vi "SaveML.vi"(6 "error in":errorcluster, 7 "Nom de la sequence":string, 8 "line":string, 9 "color win":u32(colorbox), 10 "color loose":u32(colorbox), 11 "Pos":cluster{string[], string[]}[](array[cluster])) -> (0 "error out":errorcluster, 2 "script ML":string)   [LabVIEW 2021]
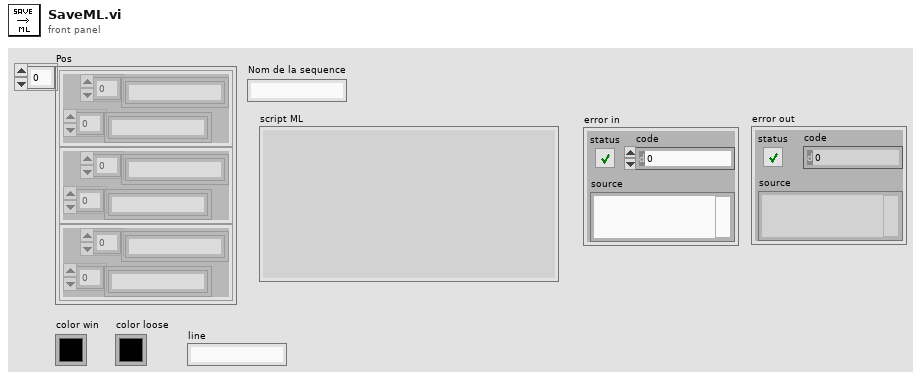
[diagram p1: front panel]
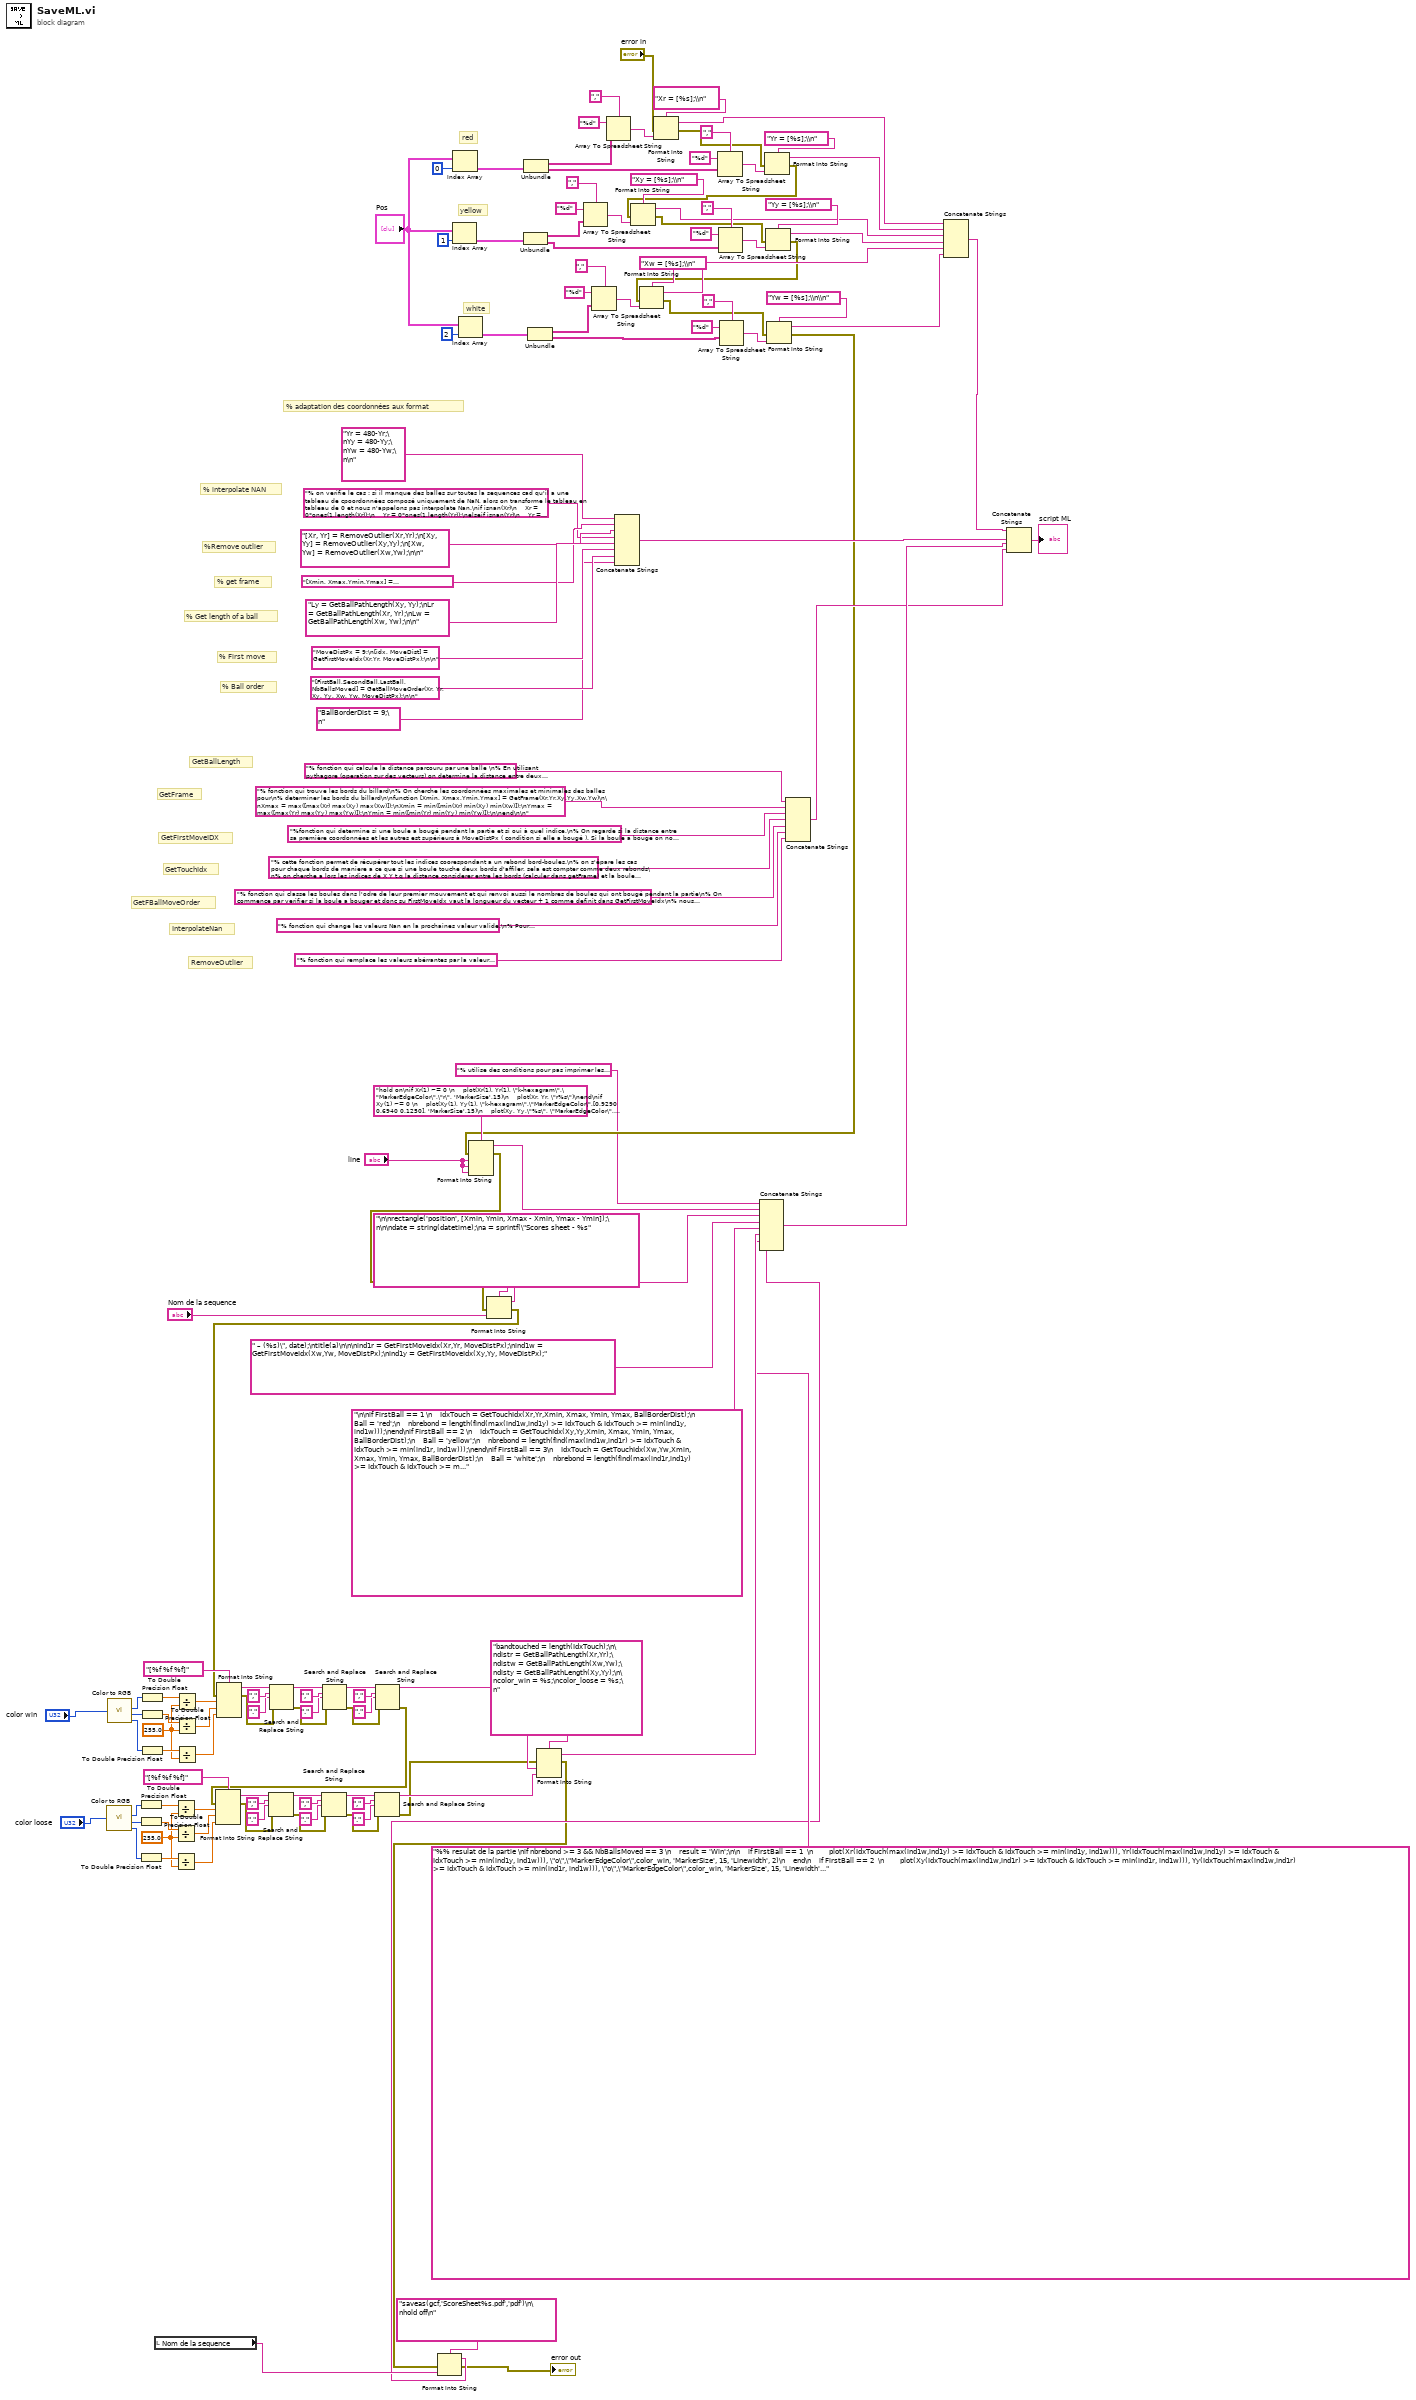
[diagram p0: block diagram]
diagram:
  w44 = 255.0
  w67 = 255.0
  # "RemoveOutlier"
  # "InterpolateNan"
  # "GetFBallMoveOrder"
  # "GetTouchIdx"
  # "GetFirstMoveIDX"
  # "GetFrame"
  # "GetBallLength"
  # "white"
  # "yellow"
  # "red"
  # "% Ball order"
  # "% First move"
  # "% Get length of a ball"
  # "% get frame"
  # "%Remove outlier"
  # "% interpolate NAN"
  # "% adaptation des coordonnées aux format"
  n1 = call <vilib>:"Color to RGB.vi"("Color"="color loose") -> ("R"=w50:u8, "G"=w49:u8, "B"=w48:u8)  [unwired: 1 out]
  n2 = call <vilib>:"Color to RGB.vi"("Color"="color win") -> ("R"=w73:u8, "G"=w72:u8, "B"=w71:u8)  [unwired: 1 out]
  n3 = To Double Precision Float(number=w50) -> (double precision float=w47:dbl)
  n4 = To Double Precision Float(number=w49) -> (double precision float=w46:dbl)
  n5 = To Double Precision Float(number=w48) -> (double precision float=w45:dbl)
  n6 = To Double Precision Float(number=w73) -> (double precision float=w70:dbl)
  n7 = To Double Precision Float(number=w72) -> (double precision float=w69:dbl)
  n8 = To Double Precision Float(number=w71) -> (double precision float=w68:dbl)
  n9 = local read "Nom de la sequence"() -> (w9:string)
  n10 = Divide(x=w47, y=w44) -> (x/y=w43:dbl)
  n11 = Divide(x=w46, y=w44) -> (x/y=w42:dbl)
  n12 = Divide(x=w45, y=w44) -> (x/y=w41:dbl)
  n13 = Divide(x=w70, y=w67) -> (x/y=w66:dbl)
  n14 = Divide(x=w69, y=w67) -> (x/y=w65:dbl)
  n15 = Divide(x=w68, y=w67) -> (x/y=w64:dbl)
  n16 = Index Array(array="Pos", index=1) -> (element=w136:cluster{string[], string[]})
  n17 = Index Array(array="Pos", index=0) -> (element=w137:cluster{string[], string[]})
  n18 = Index Array(array="Pos", index=2) -> (element=w135:cluster{string[], string[]})
  n19 = Unbundle(w136) -> (w120:string[], w106:string[])
  n20 = Unbundle(w137) -> (w134:string[], w126:string[])
  n21 = Unbundle(w135) -> (w107:string[], w105:string[])
  n22 = Array To Spreadsheet String(delimiter (Tab)=",", array=w120, 3:"%d" ("format string")) -> (spreadsheet string=w122:string)
  n23 = Array To Spreadsheet String(delimiter (Tab)=",", array=w107, 3:"%d" ("format string")) -> (spreadsheet string=w113:string)
  n24 = Array To Spreadsheet String(delimiter (Tab)=",", array=w134, 3:"%d" ("format string")) -> (spreadsheet string=w131:string)
  n25 = Concatenate Strings("Yr = 480-Yr;\nYy = 480-Yy;\nYw = 480-Yw;\n\n", "[Xmin, Xmax,Ymin,Ymax] = GetFrame(Xr,Yr,Xy,Yy,Xw,Yw);\n\n", "[Xr, Yr] = RemoveOutlier(Xr,Yr);\n[Xy, Yy] = RemoveOutlier(Xy,Yy);\n[Xw, Yw] = RemoveOutlier(Xw,Yw);\n\n", "% on verifie le cas : si il manque des balles sur toutes la sequences cad qu'il a une tableau de cpoordonnées composé uniquement de NaN, alors on transforme le tableau en tableau de 0 et nous n'appelons pas interpolate Nan.\nif isnan(Xr)\n    Xr = 0*ones(1,length(Xr));\n    Yr = 0*ones(1,length(Yr));\nelseif isnan(Yr)\n    Yr = 0*ones(1,length(Yr));\n    Xr = 0*ones(1,length(Xr));\nelse\n    [Xr, Yr] = InterpolateNan(Xr,Yr);\nend\n\nif isnan(Xy)\n    Xy = 0*ones(1,length(Xy));\n    Yy = 0*ones(1,length(Yy));\nelseif isnan(Yy)\n    Yy = 0*ones(1,length(Yy));\n    Xy = 0*ones(1,length(Xy));\nelse\n    [Xy, Yy] = InterpolateNan(Xy,Yy);\nend\n\nif isnan(Xw)\n    Xw = 0*ones(1,length(Xw));\n    Yw = 0*ones(1,length(Yw));\nelseif isnan(Yw)\n    Yw = 0*ones(1,length(Yw));\n    Xw = 0*ones(1,length(Xw));\nelse\n    [Xw, Yw] = InterpolateNan(Xw,Yw);\nend\n\n", "Ly = GetBallPathLength(Xy, Yy);\nLr = GetBallPathLength(Xr, Yr);\nLw = GetBallPathLength(Xw, Yw);\n\n", "MoveDistPx = 9;\n[idx, MoveDist] = GetFirstMoveIdx(Xr,Yr, MoveDistPx);\n\n", "[FirstBall,SecondBall,LastBall, NbBallsMoved] = GetBallMoveOrder(Xr, Yr, Xy, Yy, Xw, Yw, MoveDistPx);\n\n", "BallBorderDist = 9;\n") -> (w77:string)
  n26 = Format Into String(format string="Xr = [%s];\\n", error in="error in", w131) -> (resulting string=w87:string, error out=w25:errorcluster)  [unwired: 1 in]
  n27 = Array To Spreadsheet String(delimiter (Tab)=",", array=w126, 3:"%d" ("format string")) -> (spreadsheet string=w127:string)
  n28 = Array To Spreadsheet String(delimiter (Tab)=",", array=w106, 3:"%d" ("format string")) -> (spreadsheet string=w117:string)
  n29 = Array To Spreadsheet String(delimiter (Tab)=",", array=w105, 3:"%d" ("format string")) -> (spreadsheet string=w109:string)
  n30 = Format Into String(format string="Yr = [%s];\\n", error in=w25, w127) -> (resulting string=w104:string, error out=w24:errorcluster)  [unwired: 1 in]
  n31 = Format Into String(format string="Xy = [%s];\\n", error in=w24, w122) -> (resulting string=w103:string, error out=w23:errorcluster)  [unwired: 1 in]
  n32 = Format Into String(format string="Yy = [%s];\\n", error in=w23, w117) -> (resulting string=w102:string, error out=w22:errorcluster)  [unwired: 1 in]
  n33 = Format Into String(format string="Xw = [%s];\\n", error in=w22, w113) -> (resulting string=w101:string, error out=w21:errorcluster)  [unwired: 1 in]
  n34 = Format Into String(format string="Yw = [%s];\\n\\n", error in=w21, w109) -> (resulting string=w100:string, error out=w20:errorcluster)  [unwired: 1 in]
  n35 = Format Into String(format string="hold on\nif Xr(1) ~= 0 \n    plot(Xr(1), Yr(1), \"k-hexagram\",\"MarkerEdgeColor\",\"r\", 'MarkerSize',15)\n    plot(Xr, Yr, \"r%s\")\nend\nif Xy(1) ~= 0 \n    plot(Xy(1), Yy(1), \"k-hexagram\",\"MarkerEdgeColor\",[0.9290 0.6940 0.1250], 'MarkerSize',15)\n    plot(Xy, Yy,\"%s\", \"MarkerEdgeColor\", [0.9290 0.6940 0.1250])\nend\nif Xw(1) ~= 0 \n    plot(Xw(1), Yw(1), \"k-hexagram\",\"MarkerEdgeColor\",\"b\", 'MarkerSize',15)\n    plot(Xw, Yw, \"b%s\")\nend\n", error in=w20, "line", "line", "line") -> (resulting string=w81:string, error out=w19:errorcluster)  [unwired: 1 in]
  n36 = Format Into String(format string="\n\nrectangle('position', [Xmin, Ymin, Xmax - Xmin, Ymax - Ymin]);\n\n\ndate = string(datetime);\na = sprintf(\"Scores sheet - %s", error in=w19, "Nom de la sequence") -> (resulting string=w80:string, error out=w18:errorcluster)  [unwired: 1 in]
  n37 = Format Into String(format string="[%f %f %f]", error in=w18, w66, w65, w64) -> (resulting string=w63:string, error out=w17:errorcluster)  [unwired: 1 in]
  n38 = Search and Replace String(input string=w63, search string=",", replace string="." ("replace string (\"\")"), error in=w17) -> (result string=w56:string, error out=w16:errorcluster)  [unwired: 4 in, 2 out]
  n39 = Search and Replace String(input string=w56, search string=",", replace string="." ("replace string (\"\")"), error in=w16) -> (result string=w55:string, error out=w15:errorcluster)  [unwired: 4 in, 2 out]
  n40 = Search and Replace String(input string=w55, search string=",", replace string="." ("replace string (\"\")"), error in=w15) -> (result string=w54:string, error out=w14:errorcluster)  [unwired: 4 in, 2 out]
  n41 = Format Into String(format string="[%f %f %f]", error in=w14, w43, w42, w41) -> (resulting string=w40:string, error out=w13:errorcluster)  [unwired: 1 in]
  n42 = Search and Replace String(input string=w40, search string=",", replace string="." ("replace string (\"\")"), error in=w13) -> (result string=w33:string, error out=w12:errorcluster)  [unwired: 4 in, 2 out]
  n43 = Search and Replace String(input string=w33, search string=",", replace string="." ("replace string (\"\")"), error in=w12) -> (result string=w32:string, error out=w11:errorcluster)  [unwired: 4 in, 2 out]
  n44 = Search and Replace String(input string=w32, search string=",", replace string="." ("replace string (\"\")"), error in=w11) -> (result string=w31:string, error out=w10:errorcluster)  [unwired: 4 in, 2 out]
  n45 = Format Into String(format string="bandtouched = length(IdxTouch);\n\ndistr = GetBallPathLength(Xr,Yr);\ndistw = GetBallPathLength(Xw,Yw);\ndisty = GetBallPathLength(Xy,Yy);\n\ncolor_win = %s;\ncolor_loose = %s;\n", error in=w10, w54, w31) -> (resulting string=w30:string, error out=w6:errorcluster)  [unwired: 1 in]
  n46 = Format Into String(format string="saveas(gcf,'ScoreSheet%s.pdf','pdf')\n\nhold off\n", error in=w6, w9) -> (resulting string=w7:string, error out=→"error out":errorcluster)  [unwired: 1 in]
  n47 = Concatenate Strings("% utilise des conditions pour pas imprimer les coordonnées si la boule n'est pas la donc que sa coordonnées en X soit egale a 0\n", w81, w80, " – (%s)\", date);\ntitle(a)\n\n\nind1r = GetFirstMoveIdx(Xr,Yr, MoveDistPx);\nind1w = GetFirstMoveIdx(Xw,Yw, MoveDistPx);\nind1y = GetFirstMoveIdx(Xy,Yy, MoveDistPx);", "\n\nif FirstBall == 1 \n    IdxTouch = GetTouchIdx(Xr,Yr,Xmin, Xmax, Ymin, Ymax, BallBorderDist);\n    Ball = 'red';\n    nbrebond = length(find(max(ind1w,ind1y) >= IdxTouch & IdxTouch >= min(ind1y, ind1w)));\nend\nif FirstBall == 2 \n    IdxTouch = GetTouchIdx(Xy,Yy,Xmin, Xmax, Ymin, Ymax, BallBorderDist);\n    Ball = 'yellow';\n    nbrebond = length(find(max(ind1w,ind1r) >= IdxTouch & IdxTouch >= min(ind1r, ind1w)));\nend\nif FirstBall == 3\n    IdxTouch = GetTouchIdx(Xw,Yw,Xmin, Xmax, Ymin, Ymax, BallBorderDist);\n    Ball = 'white';\n    nbrebond = length(find(max(ind1r,ind1y) >= IdxTouch & IdxTouch >= min(ind1y, ind1r)));\nend\n", w30, "%% resulat de la partie \nif nbrebond >= 3 && NbBallsMoved == 3 \n    result = 'Win';\n\n    if FirstBall == 1  \n        plot(Xr(IdxTouch(max(ind1w,ind1y) >= IdxTouch & IdxTouch >= min(ind1y, ind1w))), Yr(IdxTouch(max(ind1w,ind1y) >= IdxTouch & IdxTouch >= min(ind1y, ind1w))), \"o\",\"MarkerEdgeColor\",color_win, 'MarkerSize', 15, 'Linewidth', 2)\n    end\n    if FirstBall == 2  \n        plot(Xy(IdxTouch(max(ind1w,ind1r) >= IdxTouch & IdxTouch >= min(ind1r, ind1w))), Yy(IdxTouch(max(ind1w,ind1r) >= IdxTouch & IdxTouch >= min(ind1r, ind1w))), \"o\",\"MarkerEdgeColor\",color_win, 'MarkerSize', 15, 'Linewidth', 2)\n    end\n    if FirstBall == 3\n        plot(Xw(IdxTouch(max(ind1r,ind1y) >= IdxTouch & IdxTouch >= min(ind1y, ind1r))), Yw(IdxTouch(max(ind1r,ind1y) >= IdxTouch & IdxTouch >= min(ind1y, ind1r))), \"o\",\"MarkerEdgeColor\",color_win, 'MarkerSize', 15, 'Linewidth', 2)\n    end\n\nelse \n    result = 'Loose';\n\n    if FirstBall == 1  \n        plot(Xr(IdxTouch), Yr(IdxTouch), \"o\",\"MarkerEdgeColor\",color_loose, 'MarkerSize', 15,  'Linewidth', 2)\n    end\n    if FirstBall == 2  \n        plot(Xy(IdxTouch), Yy(IdxTouch), \"o\",\"MarkerEdgeColor\",color_loose, 'MarkerSize', 15,  'Linewidth', 2)\n    end\n    if FirstBall == 3\n        plot(Xw(IdxTouch), Yw(IdxTouch), \"o\",\"MarkerEdgeColor\",color_loose, 'MarkerSize', 15,  'Linewidth', 2)\n    end\nend\n\n%legende \n% legend('hahahahha', 'location' , 'southeastoutside')\ntext(Xmin+20 , Ymin-10, sprintf('Score sheet for \"%s\"', Ball))\ntext(Xmin+20 , Ymin-20, sprintf('---\"%s\"---', result))\ntext(Xmin+420 , Ymin-20, sprintf('%d band(s) touched', bandtouched))\ntext(Xmin+420 , Ymin-10, sprintf('%d ball(s) moved', NbBallsMoved))\ntext(Xmin+20 , Ymin-30, sprintf('red : %.0fpx', round(distr)))\ntext(Xmin+220 , Ymin-30, sprintf('yellow : %.0f px', round(disty)))\ntext(Xmin+420 , Ymin-30, sprintf('white : %.0f px', round(distw)))\n\n \naxis off\n\n", w7) -> (w76:string)
  n48 = Concatenate Strings("% fonction qui calcule la distance parcouru par une balle \n% En utilisant pythagore (operation sur des vecteurs) on determine la distance entre deux coordonnées à l'aide de la fonction diff(X)  succésive puis on additionne ces longueurs grasse a la fct sum.\n \nfunction PathLength = GetBallPathLength(X,Y)\n\nlength_vector = sqrt(diff(X).^2 + diff(Y).^2);\nPathLength = sum(length_vector);\n\nend\n\n", "% fonction qui trouve les bords du billard\n% On cherche les coordonnées maximales et minimales des balles pour\n% determiner les bords du billard\n\nfunction [Xmin, Xmax,Ymin,Ymax] = GetFrame(Xr,Yr,Xy,Yy,Xw,Yw)\n\nXmax = max([max(Xr) max(Xy) max(Xw)]);\nXmin = min([min(Xr) min(Xy) min(Xw)]);\nYmax = max([max(Yr) max(Yy) max(Yw)]);\nYmin = min([min(Yr) min(Yy) min(Yw)]);\n\nend\n\n", "%fonction qui determine si une boule a bougé pendant la partie et si oui à quel indice.\n% On regarde si la distance entre sa première coordonnées et les autres est supérieurs à MoveDistPx ( condition si elle a bougé ). Si la boule a bougé on note l'indice de son premier mouvement dans FirstMoveIdx et la distance dans MoveDist.\n% En revanche si elle n'a pas bougé on met FirstMoveIdx au dernier indice + 1. de maniere a ce que cet indice corresponde a un indice impossible. MoveDist sera alors definit a 0.\n% De plus nous avons etudiez le cas a savoir si il manque une boule et donc que les opérations sur les vecteurs ne sont pas possibles.\nfunction [FirstMoveIdx, MoveDist] = GetFirstMoveIdx(X,Y, MoveDistPx)\nX1 = X(1);\nY1 = Y(1);\nX = X - X1;\nY = Y - Y1;\n\nif X1 == 0 && Y1 == 0\n    d = 0;\nelse\n    d = sqrt( X.^2 + Y.^2 );\nend\nif d <= MoveDistPx \n    FirstMoveIdx = length(X)+1;\n    MoveDist = 0;\nelse\n    FirstMoveIdx = find(d>MoveDistPx, 1);\n    MoveDist = sqrt(X(FirstMoveIdx).^2 + Y(FirstMoveIdx).^2);\nend\n\nend\n\n", "% cette fonction permet de récupérer tout les indices coorespondant a un rebond bord-boules.\n% on s'épare les cas pour chaque bords de maniere a ce que si une boule touche deux bords d'affiler, sela est compter comme deux rebonds\n% on cherche a lors les indices de X Y t.q la distance considerer entre les bords (calculer dans getFrame) et la boule soit inferieur ou egale a BallBorderDist.\n\nfunction [IdxTouch]=GetTouchIdx(X,Y,Xmin, Xmax, Ymin, Ymax, BallBorderDist)\n\nIdxTouch_Xmax = find( (X+BallBorderDist) >= Xmax);\nb = [0, diff(IdxTouch_Xmax)];\nIdxTouch_Xmax = IdxTouch_Xmax((b ~= 1).*IdxTouch_Xmax > 1);\n\nIdxTouch_Xmin = find( (X-BallBorderDist) <= Xmin);\nb = [0, diff(IdxTouch_Xmin)];\nIdxTouch_Xmin = IdxTouch_Xmin((b ~= 1).*IdxTouch_Xmin > 1);\n\nIdxTouch_Ymax = find( (Y+BallBorderDist) >= Ymax);\nb = [0, diff(IdxTouch_Ymax)];\nIdxTouch_Ymax = IdxTouch_Ymax((b ~= 1).*IdxTouch_Ymax > 1);\n\nIdxTouch_Ymin = find( (Y-BallBorderDist) <= Ymin);\nb = [0, diff(IdxTouch_Ymin)];\nIdxTouch_Ymin = IdxTouch_Ymin((b ~= 1).*IdxTouch_Ymin > 1);\n\nIdxTouch = sort([IdxTouch_Xmax, IdxTouch_Xmin, IdxTouch_Ymax, IdxTouch_Ymin]);\n\nend\n\n", "% fonction qui classe les boules dans l'odre de leur premier mouvement et qui renvoi aussi le nombres de boules qui ont bougé pendant la partie\n% On commence par verifier si la boule a bouger et donc su FirstMoveIdx vaut la longueur du vecteur + 1 comme definit dans GetFirstMoveIdx\n% nous cherchons donc ensuite a evaluer tout les cas possibles en commencant par chercher la plus petite de FirstMoveIdx et donc de l'appeler Firstball \n% Nous analysons ensuite la longueur de ce vecteur pour que si elle vaut 2 ou trois on comare les MoveDistPx et donc de savoir laquelle est la vrai premiere. \n% une fois que la firstball est definit, on fait de meme mais avec la plus grande Valeur de FirstMoveIdx pour definir la troisieme boules et on prossede a la meme methode que pour firstball. \n% enfin lorsque nous avons first et lastball, la deuxieme est celle qui manque et que l'on peut trouver avec la fct setdiff qui compore [lastball first ball] avec [1 2 3]\n\nfunction [FirstBall,SecondBall,LastBall, NbBallsMoved] = GetBallMoveOrder(Xr, Yr, Xy, Yy, Xw, Yw, MoveDistPx) \n\na = 3;\n\n[FirstMoveIdxr, MoveDistr] = GetFirstMoveIdx(Xr,Yr, MoveDistPx);\nif FirstMoveIdxr == length(Xr)+1\n    a = a-1;\nend\n[FirstMoveIdxy, MoveDisty] = GetFirstMoveIdx(Xy,Yy, MoveDistPx);\nif FirstMoveIdxy == length(Xy)+1\n    a = a-1;\nend\n[FirstMoveIdxw, MoveDistw] = GetFirstMoveIdx(Xw,Yw, MoveDistPx);\nif FirstMoveIdxw == length(Xw)+1\n    a = a-1;\nend\n\nNbBallsMoved = a;\n\nFirstMoveIdx = [FirstMoveIdxr, FirstMoveIdxy, FirstMoveIdxw];\nMoveDist = [MoveDistr, MoveDisty, MoveDistw];\n\nFirstBall = find(FirstMoveIdx == min(FirstMoveIdx));\n\nif length(FirstBall) == 1\n    LastBall = find(FirstMoveIdx == max(FirstMoveIdx));\n    if length(LastBall) == 2\n        LastBall = find(MoveDist == min(MoveDist(LastBall(1)), MoveDist(LastBall(2))));\n    end \nend \n\nif length(FirstBall) == 2\n    FirstBall = find(MoveDist == max(MoveDist(FirstBall(1)), MoveDist(FirstBall(2))));\n    LastBall = find(FirstMoveIdx == max(FirstMoveIdx));\nend\n\nif length(FirstBall) == 3\n    FirstBall = find(MoveDist == max(MoveDist));\n    LastBall = find(MoveDist == min(MoveDist));\nend\n\nSecondBall = setdiff([1 2 3], [FirstBall LastBall]);\n\nend\n\n", "% fonction qui change les valeurs Nan en la prochaines valeur valide.\n% Pour cela on utilise la fonction interp1.\n% On fait attention au cas ou la première valeur est un Nan car il n'est pas traité par interp1.\n\nfunction [X,Y]=InterpolateNan(X,Y)\n\nll = find(~isnan(X));\nkk = find(~isnan(Y));\nnn = find(isnan(X));\nmm = find(isnan(Y));\n\nnX = interp1([0 ll],X([1 ll]),nn,'next');\nnY = interp1([0 kk],Y([1 kk]),mm,'next');\n\nX(nn) = nX;\nY(mm) = nY;\n\nif isnan(X(1))\n    X(1)= X(2);\nend\nif isnan(Y(1))\n    Y(1)= Y(2);\nend\n\nend\n\n", "% fonction qui remplace les valeurs abérrantes par la valeur précendente.\n% Pour cela on utilise la fonction isoutlier avec la méthode movmedian.\n% Nous avons bien verifier que le outlier est bien en X et en Y.\n\nfunction [X,Y]=RemoveOutlier(X,Y)\n\nix = find(isoutlier(X,'movmedian',10));\niy = find(isoutlier(Y,'movmedian',10));\n\nidx = intersect(ix, iy);\n\nif (isempty(idx) ~=1)\n\n    if (idx(1) == 1)\n        idx=idx(2:end);\n    end\n\n    X(idx)=X(idx-1);\n    Y(idx)=Y(idx-1);\nend\n\nend \n\n") -> (w75:string)
  n49 = Concatenate Strings(w87, w104, w103, w102, w101, w100) -> (w78:string)
  n50 = Concatenate Strings(w78, w77, w76, w75) -> (→"script ML":string)
